vi "Load TSP File.vi"() -> (0 "DIMENSION":i32, 1 "Distance Opt":dbl, 2 "Tour Selection":i32[](array[numeric]), 3 "Coordinate[]":T1[](array[typedef]))   [LabVIEW 2015, in "TSP Library.lvlib"]
uses:
  TSP Library.lvlib
  TypeDef/Coordinate.ctl
panel:
  in  "Exit":bool
  in  "Load Data":bool
  out "DIMENSION Opt":i32
  out "SizeOpt IsOk":bool
  out "ParseOpt Size":i32
  in  "Opt File Path":path
  out "Parse Size":i32
  out "Size IsOk":bool
  in  "TSP File Path":path
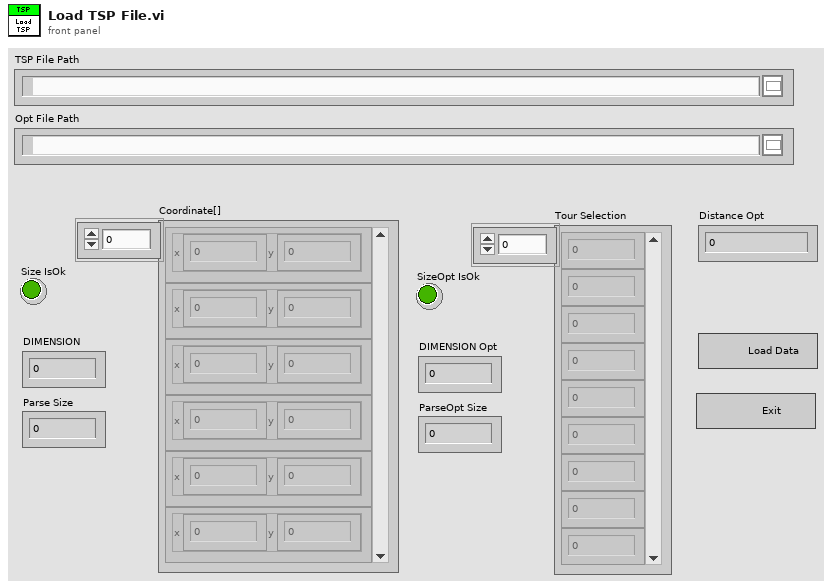
[diagram p1: front panel]
types:
  T1 = typedef "TSP Library.lvlib/Coordinate.ctl" = cluster{"x":dbl, "y":dbl}
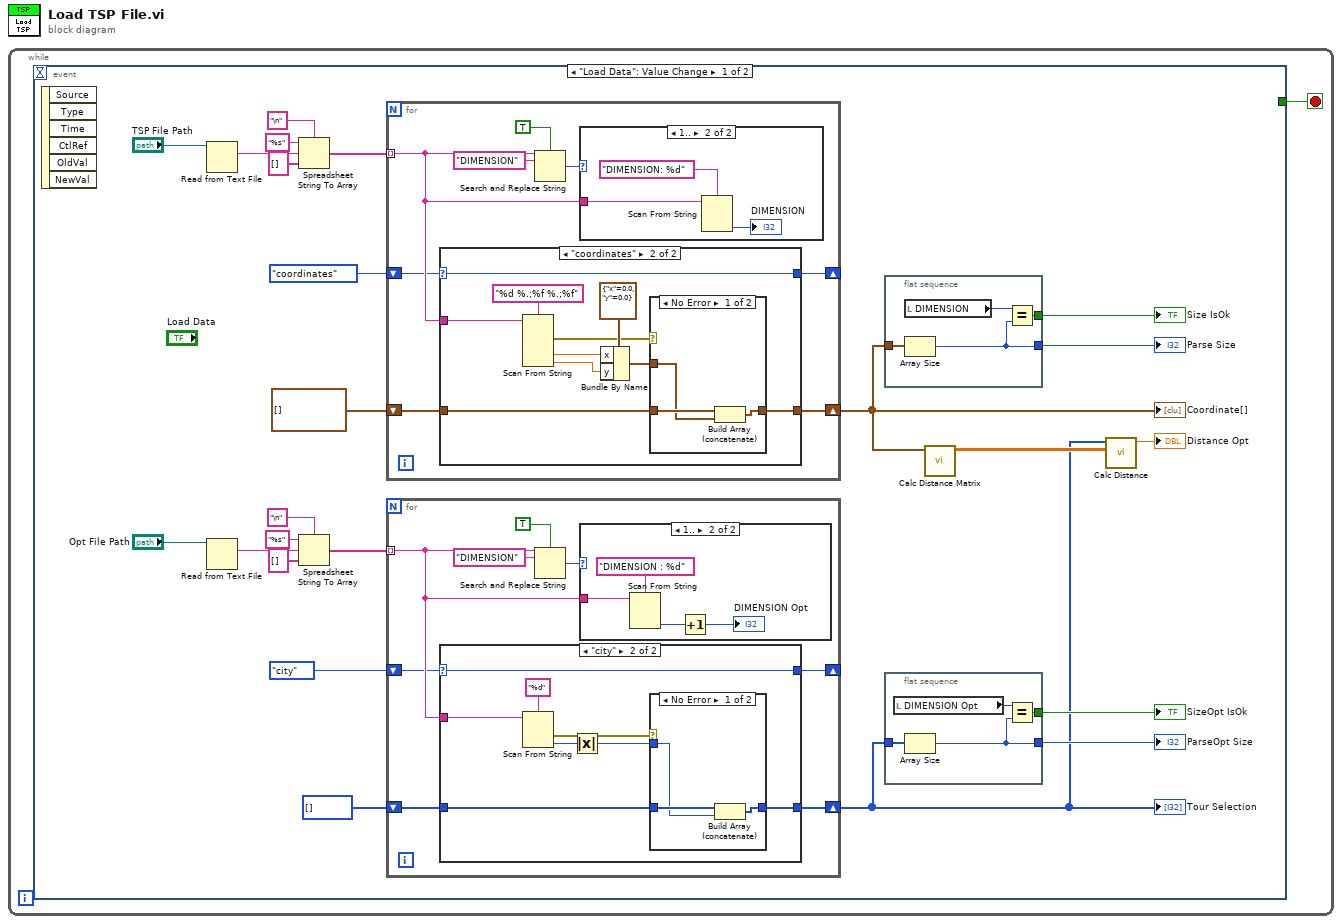
[diagram p0: block diagram]
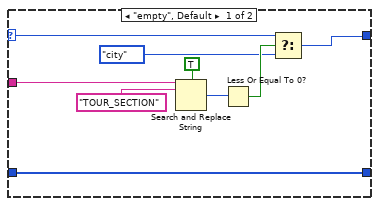
[diagram p2: hidden frame]
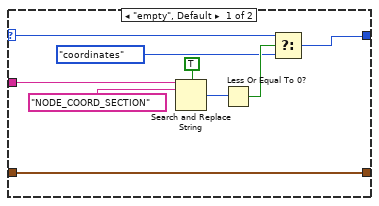
[diagram p5: hidden frame]
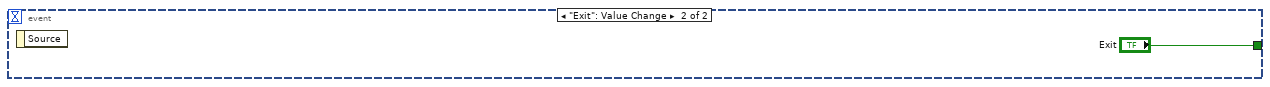
[diagram p8: hidden frame]
diagram:
  n1 = while {
    stop <- w1 stop-if-true
    n2 = event shown="[0] \"Load Data\": Value Change" {
      selector: _ -> [_ _]
      dyn-events: _ -> [_ _]
      timeout: _ -> [_ _]
      tunnel: [_ "Exit"] -> w1
      event "Load Data": Value Change {
        n3 = event-data() -> ()  [unwired: 1 in, 6 out]
        n4 = Read from Text File(file (use dialog)="TSP File Path") -> (text=w24:string)  [unwired: 3 in, 3 out]
        n5 = Read from Text File(file (use dialog)="Opt File Path") -> (text=w7:string)  [unwired: 3 in, 3 out]
        n6 = Spreadsheet String To Array(delimiter (Tab)="\n", format string="%s", spreadsheet string=w24, array type (2D Dbl)=string[] []) -> (array=w20:string[])
        n7 = Spreadsheet String To Array(delimiter (Tab)="\n", format string="%s", spreadsheet string=w7, array type (2D Dbl)=string[] []) -> (array=w11:string[])
        n8 = for {
          tunnel: w20 -> [w71] mode=indexing
          shift-right: [w69] -> _
          shift-left: enum16{"empty", "coordinates"}."coordinates" -> [w70]
          shift-right: [w67] -> w4
          shift-left: T1[] [] ("Array") -> [w68]
          n9 = case shown="\"coordinates\"" w70 {
            selector: w70 -> [w78 w93]
            tunnel: w71 -> [w81 w92]
            tunnel: [w77 w93] -> w69
            tunnel: w68 -> [w75 w86]
            tunnel: [w75 w85] -> w67
            frame "empty", Default {
              n10 = Search and Replace String(case sensitive?=TRUE ("ignore case? (F)"), input string=w81, search string="NODE_COORD_SECTION") -> (number of replacements=w80:i32)  [unwired: 5 in, 3 out]
              n11 = Less Or Equal To 0?(x=w80) -> (x <= 0?=w79:bool)
              n12 = Select(t=w78, s=w79, f=enum16{"empty", "coordinates"}."coordinates") -> (s? t:f=w77:enum16{"empty", "coordinates"})
            }
            frame "coordinates" {
              n13 = Scan From String(format string="%d %.;%f %.;%f", input string=w92) -> (error out=w87:errorcluster, output 2=w89:dbl, output 3=w88:dbl)  [unwired: 6 in, 2 out]
              n14 = Bundle By Name(cluster=T1 {"x"=0.0, "y"=0.0} ("Coordinate"), "x"=w89, "y"=w88) -> (w84:T1)
              n15 = case shown="No Error" w87 {
                tunnel: [w95 w97] -> w85
                tunnel: w86 -> [w96 w97]
                tunnel: w84 -> [w94 _]
                frame No Error {
                  n16 = Build Array (concatenate)(w96, w94) -> (w95:T1[])
                }
                frame Error {
                }
              }
            }
          }
          n17 = Search and Replace String(case sensitive?=TRUE ("ignore case? (F)"), input string=w71, search string="DIMENSION") -> (number of replacements=w72:i32)  [unwired: 5 in, 3 out]
          n18 = case shown="1.." w72 {
            tunnel: w71 -> [_ w100]
            frame ..0, Default {
            }
            frame 1.. {
              n19 = Scan From String(format string="DIMENSION: %d", input string=w100) -> (output 1=→"DIMENSION":i32)  [unwired: 3 in, 3 out]
            }
          }
        }
        "Coordinate[]" <- w4
        n20 = for {
          tunnel: w11 -> [w34] mode=indexing
          shift-right: [w32] -> _
          shift-left: enum16{"empty", "city"}."city" -> [w33]
          shift-right: [w30] -> w2
          shift-left: i32[] [] ("Array") -> [w31]
          n21 = case shown="\"city\"" w33 {
            selector: w33 -> [w41 w54]
            tunnel: w34 -> [w44 w53]
            tunnel: [w40 w54] -> w32
            tunnel: w31 -> [w38 w50]
            tunnel: [w38 w49] -> w30
            frame "empty", Default {
              n22 = Search and Replace String(case sensitive?=TRUE ("ignore case? (F)"), input string=w44, search string="TOUR_SECTION") -> (number of replacements=w43:i32)  [unwired: 5 in, 3 out]
              n23 = Less Or Equal To 0?(x=w43) -> (x <= 0?=w42:bool)
              n24 = Select(t=w41, s=w42, f=enum16{"empty", "city"}."city") -> (s? t:f=w40:enum16{"empty", "city"})
            }
            frame "city" {
              n25 = Scan From String(format string="%d", input string=w53) -> (error out=w51:errorcluster, output 1=w48:i32)  [unwired: 3 in, 2 out]
              n26 = Absolute Value(x=w48) -> (abs(x)=w47:i32)
              n27 = case shown="No Error" w51 {
                tunnel: [w56 w58] -> w49
                tunnel: w50 -> [w57 w58]
                tunnel: w47 -> [w55 _]
                frame No Error {
                  n28 = Build Array (concatenate)(w57, w55) -> (w56:i32[])
                }
                frame Error {
                }
              }
            }
          }
          n29 = Search and Replace String(case sensitive?=TRUE ("ignore case? (F)"), input string=w34, search string="DIMENSION") -> (number of replacements=w35:i32)  [unwired: 5 in, 3 out]
          n30 = case shown="1.." w35 {
            tunnel: w34 -> [_ w62]
            frame ..0, Default {
            }
            frame 1.. {
              n31 = Scan From String(format string="DIMENSION : %d", input string=w62) -> (output 1=w60:i32)  [unwired: 3 in, 3 out]
              n32 = Increment(x=w60) -> (x+1=→"DIMENSION Opt":i32)
            }
          }
        }
        "Tour Selection" <- w2
        n33 = flat-sequence {
          tunnel: w4 -> [w66]
          tunnel: [w64] -> w17
          tunnel: [w63] -> w16
          frame #0 {
            n34 = local read "DIMENSION"() -> (w65:i32)
            n35 = Array Size(array=w66) -> (size(s)=w63:i32)
            n36 = Equal?(x=w65, y=w63) -> (x = y?=w64:bool)
          }
        }
        n37 = flat-sequence {
          tunnel: w2 -> [w29]
          tunnel: [w27] -> w14
          tunnel: [w26] -> w15
          frame #0 {
            n38 = local read "DIMENSION Opt"() -> (w28:i32)
            n39 = Array Size(array=w29) -> (size(s)=w26:i32)
            n40 = Equal?(x=w28, y=w26) -> (x = y?=w27:bool)
          }
        }
        n41 = call "Calc Distance Matrix.vi"("Coordinate[]"=w4) -> ("Distance Matrix"=w3:dbl[][])  [unwired: 10 in]
        n42 = call "Calc Distance.vi"("Distance Matrix"=w3, "Tour"=w2) -> ("Distance"=→"Distance Opt":dbl)  [unwired: 9 in]
        "Size IsOk" <- w17
        "Parse Size" <- w16
        "SizeOpt IsOk" <- w14
        "ParseOpt Size" <- w15
      }
      event "Exit": Value Change {
        n43 = event-data() -> ()  [unwired: 1 in, 1 out]
      }
    }
  }
